vi "[FGV] Overlay.vi"(7 "Enum":enum16{"initialize", "Original Image", "Read"}(ring), 8 "error in (no error)":errorcluster, 11 "Image":T1) -> (0 "error out":errorcluster, 3 "Vision_Image":T1(plugin-control))   [LabVIEW 2015]
uses:
  <vilib>/vision/Image Controls.llb/IMAQ Image.ctl
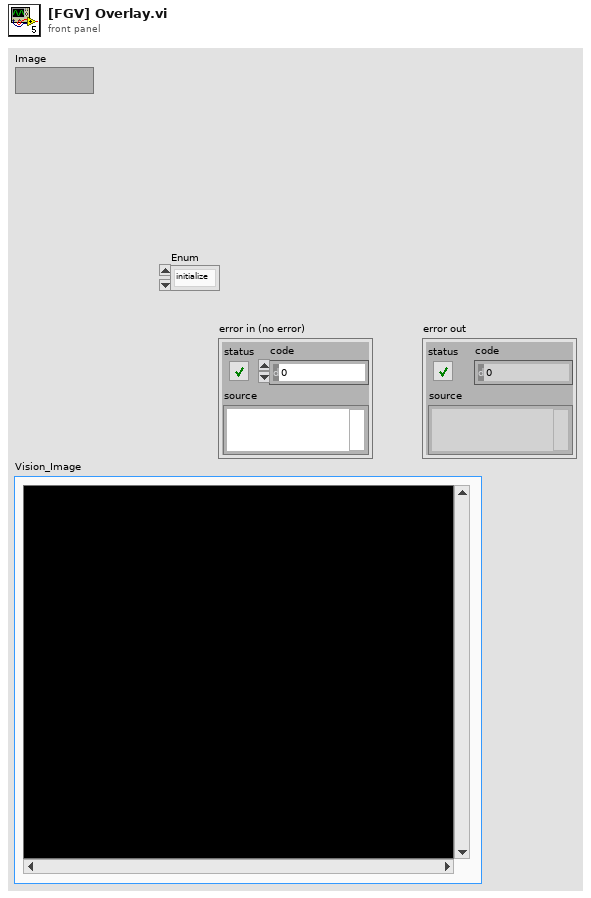
[diagram p1: front panel]
types:
  T1 = typedef "IMAQ Image.ctl" = refnum<image>
  T2 = typedef "Image Type" = u32
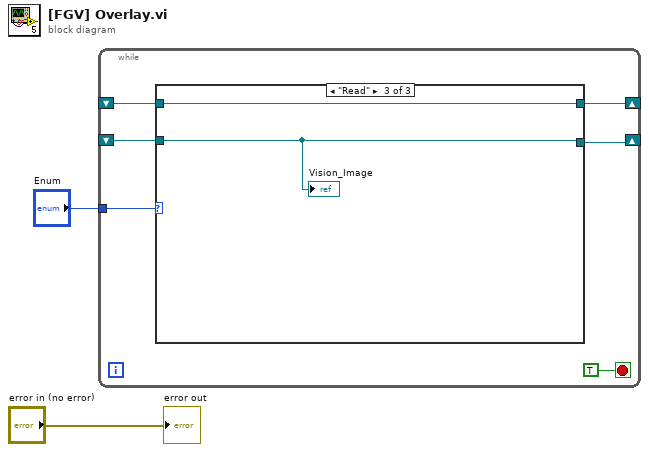
[diagram p0: block diagram]
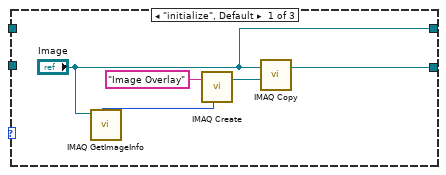
[diagram p2: hidden frame]
diagram:
  n1 = while {
    tunnel: "Enum" -> [w7]
    shift-right: [w6] -> _
    shift-left: _ -> [w5]
    shift-right: [w4] -> _
    shift-left: _ -> [w3]
    stop <- TRUE stop-if-true
    n2 = case shown="\"Read\"" w7 {
      tunnel: [w11 w14 w15] -> w6
      tunnel: w5 -> [_ _ w15]
      tunnel: ["Image" w14 w16] -> w4
      tunnel: w3 -> [_ w14 w16]
      frame "initialize", Default {
        n3 = call "IMAQ GetImageInfo"("Image"="Image") -> ("Image Type"=w10:T2)  [unwired: 3 in, 7 out]
        n4 = call "IMAQ Create"("Image Name"="Image Overlay", "Image Type"=w10) -> ("New Image"=w13:T1)  [unwired: 3 in, 1 out]
        n5 = call "IMAQ Copy"("Image Dst"=w13, "Image Src"="Image") -> ("Image Dst Out"=w11:T1)  [unwired: 4 in, 1 out]
      }
      frame "Original Image" {
      }
      frame "Read" {
        "Vision_Image" <- w15
      }
    }
  }
  "error out" <- "error in (no error)"
